vi "Digilens DLP Gen2 UI .vi"(11 "TopLevel In":refnum<class "TopLevel.lvclass">) -> (3 "TopLevel Out":refnum<class "TopLevel.lvclass">)   [LabVIEW 2022 SP3, in "TopLevel.lvclass"] (continued)
            n239 = call <vilib>:"Add State(s) to Queue__JKI_lib_State_Machine.vi"("State(s) in Front (\"\")"="UI: CheckConfigRequired\nUI: UpatePrinterPage" ("State(s) in Front (\"\")"), "State(s) in (\"\")"=w621) -> ("States Out"=w620:string)  [unwired: 13 in]
          }
          event User Event {
            (unwired) "Data: Verify Materials and Color planes" ("State(s) in Front (\"\")")
            n240 = event-data() -> ("Paths"=w660:T36, "ColorPaneMapping"=w659:T37)  [unwired: 1 in, 4 out]
            n241 = Bundle By Name(cluster=w663, "DLP2Config.Paths"=w660, "DLP2Config.ColorPaneMapping"=w659) -> (w661:T77)
            n242 = call <vilib>:"Add State(s) to Queue__JKI_lib_State_Machine.vi"("State(s) in (\"\")"=w666) -> ("States Out"=w665:string)  [unwired: 14 in]
          }
          event "Apply DLP GUI Config": Value Change {
            # "Note: Cannot be blocking"
            n243 = event-data() -> ()  [unwired: 1 in, 6 out]
            n244 = call-dynamic "ApplyDLP2GUIConfig_API.vi"("error in (no error)"=w668, "DLP GUI Config"="DLP GUI Config", "TopLevel in"=w670) -> ("error out"=w669:errorcluster, "TopLevel out"=w671:refnum<class "TopLevel.lvclass">)  [unwired: 7 in]
            n245 = call <vilib>:"Add State(s) to Queue__JKI_lib_State_Machine.vi"("State(s) in (\"\")"=w674) -> ("States Out"=w673:string)  [unwired: 14 in]
          }
          event "SAVE DLP Config": Value Change {
            n246 = event-data() -> ()  [unwired: 1 in, 6 out]
            n247 = Unbundle By Name(w685) -> ("TopLevel out"=w684:refnum<class "TopLevel.lvclass">, "DLP2Config"=w676:T35)
            n248 = call-dynamic "Write Digilens Config 2.vi"("error in (no error)"=w683, "MasterConfigurationDLPC2"=w676, "TopLevel in"=w684) -> ("error out"=w679:errorcluster, "TopLevel out"=w681:refnum<class "TopLevel.lvclass">)  [unwired: 7 in]
            n249 = property on="DLP GUI Config" class="Path"(error in=w679) -> (error out=w680:errorcluster, "Value"=w682:path)  [unwired: 1 in, 1 out]
            n250 = call-dynamic "SaveDLP2GUIConfig_API.vi"("error in (no error)"=w680, "DLP GUI Config"=w682, "TopLevel in"=w681) -> ("error out"=w678:errorcluster)  [unwired: 7 in, 1 out]
            n251 = Bundle By Name(cluster=w685, "DLP2ConfigLoaded"=w676, "ConfigSaveRequired"=FALSE) -> (w677:T77)
            n252 = call <vilib>:"Add State(s) to Queue__JKI_lib_State_Machine.vi"("State(s) in (\"\")"=w688) -> ("States Out"=w687:string)  [unwired: 14 in]
          }
          event "GetMat&Color": Value Change {
            n253 = event-data() -> ()  [unwired: 1 in, 6 out]
            n254 = call <vilib>:"Add State(s) to Queue__JKI_lib_State_Machine.vi"("State(s) in Front (\"\")"="Data: GetMaterialsAndColorPlanes" ("State(s) in Front (\"\")"), "State(s) in (\"\")"=w694) -> ("States Out"=w693:string)  [unwired: 13 in]
          }
          event User Event {
            n255 = event-data() -> ("PrintNo"=→"Print #":i32, "PrePurgePrintNo"=→"Counts":i32, "CalPrintNo"=→"CalPrint Counter":i32)  [unwired: 1 in, 7 out]
            n256 = call <vilib>:"Add State(s) to Queue__JKI_lib_State_Machine.vi"("State(s) in Front (\"\")"="UI: Update Stage Busy" ("State(s) in Front (\"\")"), "State(s) in (\"\")"=w703) -> ("States Out"=w702:string)  [unwired: 13 in]
          }
          event "Abort", "AbortPrinterOperation", "Abort 2": Value Change {
            n257 = event-data() -> ()  [unwired: 1 in, 6 out]
            n258 = Unbundle By Name(w718) -> ("TopLevel out"=w707:refnum<class "TopLevel.lvclass">, "Motor Controller"=w715:refnum<class "Motor Controller.lvclass">, "GIS Printer"=w709:refnum<class "GIS Printer.lvclass">)
            n259 = call-dynamic "Abort API.vi"("error in (no error)"=w705, "TopLevel in"=w707) -> ("error out"=w706:errorcluster)  [unwired: 8 in, 1 out]
            n260 = call "Generate Abort Event GIS Printer.vi"("error in (no error)"=w706, "GIS Printer in"=w709) -> ("error out"=w710:errorcluster, "GIS Printer out"=w708:refnum<class "GIS Printer.lvclass">)  [unwired: 8 in]
            n261 = disable-structure shown="Enabled" {
              disable-tunnel: "AbortPrint" ("Task ID") -> [w726 _]
              disable-tunnel: FALSE ("Wait (F)") -> [w725 _]
              disable-tunnel: [w724 w727] -> w712
              disable-tunnel: w708 -> [w723 _]
              disable-tunnel: w710 -> [w722 w727]
              frame Disabled {
                n262 = call "API_Abort.vi"("Wait (F)"=w725, "error in (no error)"=w722, "Task ID"=w726, "GIS Printer in"=w723) -> ("error out"=w724:errorcluster)  [unwired: 5 in, 2 out]
              }
              frame Enabled {
              }
            }
            n263 = call "API_AbortStage.vi"("Wait (F)"=FALSE, "error in (no error)"=w712, "Task ID"="AbortMotor", "Motor Controller in"=w715) -> ("error out"=w711:errorcluster)  [unwired: 5 in, 2 out]
            n264 = call <vilib>:"Add State(s) to Queue__JKI_lib_State_Machine.vi"("State(s) in Front (\"\")"="UI: Update Status>>Abort" ("State(s) in Front (\"\")"), "State(s) in (\"\")"=w721) -> ("States Out"=w720:string)  [unwired: 13 in]
          }
          event "Stage Abort": Value Change {
            n265 = event-data() -> ()  [unwired: 1 in, 6 out]
            n266 = Unbundle By Name(w733) -> ("Motor Controller"=w732:refnum<class "Motor Controller.lvclass">)  [unwired: 1 out]
            n267 = call "API_AbortStage.vi"("Wait (F)"=FALSE, "error in (no error)"=w728, "Task ID"="AbortMotor", "Motor Controller in"=w732) -> ("error out"=w729:errorcluster)  [unwired: 5 in, 2 out]
            n268 = call <vilib>:"Add State(s) to Queue__JKI_lib_State_Machine.vi"("State(s) in (\"\")"=w736) -> ("States Out"=w735:string)  [unwired: 14 in]
          }
          event Panel Close? {
            # "Discard the event because we'll close the front panel ourselves in Macro: Exit"
            n269 = event-data() -> ()  [unwired: 1 in, 1 out]
            n270 = event-data("Discard?"=TRUE) -> ()  [unwired: 1 in, 1 out]
            n271 = call <vilib>:"Add State(s) to Queue__JKI_lib_State_Machine.vi"("State(s) in Front (\"\")"="Macro: Exit", "State(s) in (\"\")"=w743) -> ("States Out"=w742:string)  [unwired: 13 in]
          }
          event "Exit": Value Change {
            n272 = event-data() -> ()  [unwired: 1 in, 6 out]
            n273 = Two Button Dialog(message="Are you sure you want to Exit the Application?", 2:"Exit" ("T button name (\"OK\")")) -> (T button?=w747:bool)  [unwired: 1 in]
            n274 = Select(t="Macro: Exit", s=w747, f="") -> (s? t:f=w744:string)
            n275 = call <vilib>:"Add State(s) to Queue__JKI_lib_State_Machine.vi"("State(s) in Front (\"\")"=w744, "State(s) in (\"\")"=w754) -> ("States Out"=w753:string)  [unwired: 13 in]
          }
          event User Event {
            n276 = event-data() -> ("Motor Controller Config Data"=w763:T41, "Motor Controller Data"=w762:cluster{"Enabled?":bool}, "Stage Move.Current Step"=→"Status":string, "Stage Move.Move Data"=w761:T43[], "Stage Busy?"=w755:bool)  [unwired: 1 in, 4 out]
            n277 = flat-sequence {
              tunnel: w755 -> [_]
              frame #0 {
              }
            }
            n278 = Unbundle By Name(w763) -> ("Current Position"=→"Position":i32, "Pulse_Per_mm"=→"Pulse/mm":i32, "PrePrint"=w771:dbl[])
            n279 = Unbundle By Name(w762) -> ()  [unwired: 1 out]
            n280 = Bundle By Name(cluster=w775, "Status.Motor Controller Config Data"=w763, "Status.Motor Controller Data"=w762) -> (w764:T77)
            n281 = for {
              tunnel: w761 -> [w784] mode=indexing
              tunnel: [w777] -> w759 mode=indexing
              n282 = Unbundle By Name(w784) -> ("Move.Index_mm"=w783:i32, "Move.Speed_mm_s"=w782:i32, "Status"=w779:T44)
              n283 = Format Into String(w783) -> (resulting string=w781:string)  [unwired: 3 in, 1 out]
              n284 = Format Into String(w782) -> (resulting string=w780:string)  [unwired: 3 in, 1 out]
              n285 = Format Into String(w779) -> (resulting string=w778:string)  [unwired: 3 in, 1 out]
              n286 = Build Array(w781, w780, w778) -> (w777:string[])
            }
            n287 = Index Array(array=w771) -> (element #1=→"H1":dbl, element #2=→"H 2":dbl, element #3=→"H 3":dbl, element #4=→"H 4":dbl, element #5=→"H 5":dbl, element #6=→"H 6":dbl)  [unwired: 6 in]
            n288 = property on="Stage Move Status" class="MCListbox (strict)"("ItemNames"=w759) -> ()  [unwired: 2 in, 2 out]
            n289 = call <vilib>:"Add State(s) to Queue__JKI_lib_State_Machine.vi"("State(s) in Front (\"\")"="UI: Update Stage Busy", "State(s) in (\"\")"=w757) -> ("States Out"=w758:string)  [unwired: 13 in]
          }
          event User Event {
            n290 = event-data() -> ("UsrEvtRef"=w790:refnum<user-event>)  [unwired: 1 in, 3 out]
            n291 = Flush Event Queue(0:w791, 2:w790, 3:w786, 5:1 ("keep most recent")) -> (8:w788:refnum<event-registration>, 11:w787:errorcluster)  [unwired: 2 in, 1 out]
            n292 = call <vilib>:"Add State(s) to Queue__JKI_lib_State_Machine.vi"("State(s) in Front (\"\")"="DI: Get ICP2 DI Status\nDO: Set ICP1-DO Status in UI\nDO: Set ICP2-DO Status in UI\nAI: Get ICP1 AI Status\nAO: Set ICP1-AO Status in UI\nAO: Set ICP2-AO Status in UI" ("State(s) in Front (\"\")"), "State(s) in (\"\")"=w792) -> ("States Out"=w793:string)  [unwired: 13 in]
          }
          event Value Change {
            n293 = event-data() -> ()  [unwired: 1 in, 6 out]
            n294 = case shown="True" "Enable Disable" {
              tunnel: [Motor_Controller_Parameter-Set."Enable Servo" ("Motor Controller Parameter") Motor_Controller_Parameter-Set."Disable Servo" ("Motor Controller Parameter")] -> w807
              tunnel: [1 ("value") 0 ("value")] -> w804
              frame True {
              }
              frame False {
              }
            }
            n295 = Bundle By Name(cluster=T20 {"Motor Controller Parameter"=enum."Print Speed", "value"=0} ("SetExplicitMessage API Data"), "Motor Controller Parameter"=w807, "value"=w804) -> (w806:T20)
            n296 = Unbundle By Name(w801) -> ("Motor Controller"=w812:refnum<class "Motor Controller.lvclass">)
            n297 = Bundle By Name(cluster=T23 {"Command"=enum."GetExplicitMessage", "Arguments"="", "Data"=variant} ("API Command Cluster"), "Command"=API_Command_Enum."SetExplicitMessage", "Data"=w806) -> (w805:T23)
            n298 = call-dynamic "GenerateAPIEvent_Motor Controller.vi"("error in (no error)"=w811, "API Command Cluster"=w805, "Motor Controller In"=w812) -> ("error out"=w798:errorcluster)  [unwired: 6 in, 2 out]
            n299 = Unbundle By Name(w801) -> ("DAQ"=w802:refnum<class "DAQ.lvclass">)
            n300 = Format Into String(format string="%s", ICP1-D0_Channel_Names."Servo ON" ("DO Channel")) -> (resulting string=w800:string)  [unwired: 2 in, 1 out]
            n301 = call "Set DO State (manual mode).vi"("error in (no error)"=w798, "State"="Enable Disable", "DO IOName"=w800, "DAQ"=w802) -> ("error out"=w797:errorcluster)  [unwired: 6 in, 1 out]
          }
          event "5Pass": Value Change {
            n302 = event-data() -> ()  [unwired: 1 in, 6 out]
            n303 = Bundle By Name(cluster=T20 {"Motor Controller Parameter"=enum."Print Speed", "value"=0} ("SetExplicitMessage API Data"), "Motor Controller Parameter"=Motor_Controller_Parameter-Set."PR Path", "value"=20) -> (w821:T20)
            n304 = Unbundle By Name(w829) -> ("Motor Controller"=w828:refnum<class "Motor Controller.lvclass">)
            n305 = Bundle By Name(cluster=T23 {"Command"=enum."GetExplicitMessage", "Arguments"="", "Data"=variant} ("API Command Cluster"), "Command"=API_Command_Enum."SetExplicitMessage", "Data"=w821) -> (w820:T23)
            n306 = call-dynamic "GenerateAPIEvent_Motor Controller.vi"("error in (no error)"=w826, "API Command Cluster"=w820, "Motor Controller In"=w828) -> ("error out"=w827:errorcluster)  [unwired: 6 in, 2 out]
          }
          event "10Pass": Value Change {
            n307 = event-data() -> ()  [unwired: 1 in, 6 out]
            n308 = Bundle By Name(cluster=T20 {"Motor Controller Parameter"=enum."Print Speed", "value"=0} ("SetExplicitMessage API Data"), "Motor Controller Parameter"=Motor_Controller_Parameter-Set."PR Path", "value"=30) -> (w834:T20)
            n309 = Unbundle By Name(w842) -> ("Motor Controller"=w841:refnum<class "Motor Controller.lvclass">)
            n310 = Bundle By Name(cluster=T23 {"Command"=enum."GetExplicitMessage", "Arguments"="", "Data"=variant} ("API Command Cluster"), "Command"=API_Command_Enum."SetExplicitMessage", "Data"=w834) -> (w833:T23)
            n311 = call-dynamic "GenerateAPIEvent_Motor Controller.vi"("error in (no error)"=w839, "API Command Cluster"=w833, "Motor Controller In"=w841) -> ("error out"=w840:errorcluster)  [unwired: 6 in, 2 out]
          }
          event Value Change {
            n312 = event-data() -> ("CtlRef"=w847:refnum<vi>)  [unwired: 1 in, 5 out]
            n313 = property class="Bool"(reference=w847) -> ("Label.Text"=w846:string)  [unwired: 1 in, 2 out]
            n314 = case shown="\"Head6\"" w846 {
              tunnel: [Motor_Controller_Parameter-Set."Move Stage to Under PH1" ("Motor Controller Parameter") Motor_Controller_Parameter-Set."Move Stage to Under PH1" ("Motor Controller Parameter") Motor_Controller_Parameter-Set."Move Stage to Under PH2" ("Motor Controller Parameter") Motor_Controller_Parameter-Set."Move Stage to Under PH2" ("Motor Controller Parameter") Motor_Controller_Parameter-Set."Move Stage to Under PH3" ("Motor Controller Parameter") Motor_Controller_Parameter-Set."Move Stage to Under PH3" ("Motor Controller Parameter") Motor_Controller_Parameter-Set."Move Stage to Under PH4" ("Motor Controller Parameter") Motor_Controller_Parameter-Set."Move Stage to Under PH4" ("Motor Controller Parameter") Motor_Controller_Parameter-Set."Move Stage to Under PH5" ("Motor Controller Parameter") Motor_Controller_Parameter-Set."Move Stage to Under PH5" ("Motor Controller Parameter") Motor_Controller_Parameter-Set."Move Stage to Under PH6" ("Motor Controller Parameter") Motor_Controller_Parameter-Set."Move Stage to Under PH6" ("Motor Controller Parameter")] -> w849
              tunnel: [11 ("value") 4 ("value") 12 ("value") 5 ("value") 13 ("value") 6 ("value") 14 ("value") 7 ("value") 15 ("value") 8 ("value") 16 ("value") 9 ("value")] -> w848
              frame "Head1", Default {
              }
              frame "PurgeMove H1" {
              }
              frame "Head2" {
              }
              frame "PurgeMove H2" {
              }
              frame "Head3" {
              }
              frame "PurgeMove H3" {
              }
              frame "Head4" {
              }
              frame "PurgeMove H4" {
              }
              frame "Head5" {
              }
              frame "PurgeMove H5" {
              }
              frame "Head6" {
              }
              frame "PurgeMove H6" {
              }
            }
            n315 = Bundle By Name(cluster=T20 {"Motor Controller Parameter"=enum."Move Stage to Under PH1", "value"=11} ("SetExplicitMessage API Data"), "value"=w848, "Motor Controller Parameter"=w849) -> (w845:T20)
            n316 = Unbundle By Name(w853) -> ("Motor Controller"=w857:refnum<class "Motor Controller.lvclass">)
            n317 = Bundle By Name(cluster=T23 {"Command"=enum."GetExplicitMessage", "Arguments"="", "Data"=variant} ("API Command Cluster"), "Command"=API_Command_Enum."SetExplicitMessage", "Data"=w845) -> (w854:T23)
            n318 = call-dynamic "GenerateAPIEvent_Motor Controller.vi"("error in (no error)"=w851, "API Command Cluster"=w854, "Motor Controller In"=w857) -> ("error out"=w852:errorcluster)  [unwired: 6 in, 2 out]
          }
          event "Heater-1 Off 2": Value Change {
            n319 = event-data() -> ("NewVal"=w884:bool)  [unwired: 1 in, 5 out]
            n320 = Bundle By Name(cluster=w891, "Heater Enable.HeaterEnblHead"=PrinterHeads--Enum."1" ("Heater Enable.Head"), "Heater Enable.Enable"=w884, "PersistentData.HeatEnable.Heater-1 Off"=w884) -> (w889:T77)
            n321 = call <vilib>:"Add State(s) to Queue__JKI_lib_State_Machine.vi"("State(s) in Front (\"\")"="Heater: Enable Disable\nData: Write to Persistent File", "State(s) in (\"\")"=w886) -> ("States Out"=w887:string)  [unwired: 13 in]
          }
          event "Heater-2 Off 2": Value Change {
            n322 = event-data() -> ("NewVal"=w893:bool)  [unwired: 1 in, 5 out]
            n323 = Bundle By Name(cluster=w900, "Heater Enable.HeaterEnblHead"=PrinterHeads--Enum."2" ("Heater Enable.Head"), "Heater Enable.Enable"=w893, "PersistentData.HeatEnable.Heater-2 Off"=w893) -> (w898:T77)
            n324 = call <vilib>:"Add State(s) to Queue__JKI_lib_State_Machine.vi"("State(s) in Front (\"\")"="Heater: Enable Disable\nData: Write to Persistent File", "State(s) in (\"\")"=w895) -> ("States Out"=w896:string)  [unwired: 13 in]
          }
          event "Heater-3 Off 2": Value Change {
            n325 = event-data() -> ("NewVal"=w902:bool)  [unwired: 1 in, 5 out]
            n326 = Bundle By Name(cluster=w909, "Heater Enable.HeaterEnblHead"=PrinterHeads--Enum."3" ("Heater Enable.Head"), "Heater Enable.Enable"=w902, "PersistentData.HeatEnable.Heater-3 Off"=w902) -> (w907:T77)
            n327 = call <vilib>:"Add State(s) to Queue__JKI_lib_State_Machine.vi"("State(s) in Front (\"\")"="Heater: Enable Disable\nData: Write to Persistent File", "State(s) in (\"\")"=w904) -> ("States Out"=w905:string)  [unwired: 13 in]
          }
          event "Heater-4 Off 2": Value Change {
            n328 = event-data() -> ("NewVal"=w911:bool)  [unwired: 1 in, 5 out]
            n329 = Bundle By Name(cluster=w918, "Heater Enable.HeaterEnblHead"=PrinterHeads--Enum."4" ("Heater Enable.Head"), "Heater Enable.Enable"=w911, "PersistentData.HeatEnable.Heater-4 Off"=w911) -> (w916:T77)
            n330 = call <vilib>:"Add State(s) to Queue__JKI_lib_State_Machine.vi"("State(s) in Front (\"\")"="Heater: Enable Disable\nData: Write to Persistent File", "State(s) in (\"\")"=w913) -> ("States Out"=w914:string)  [unwired: 13 in]
          }
          event "Heater-5 Off 2": Value Change {
            n331 = event-data() -> ("NewVal"=w920:bool)  [unwired: 1 in, 5 out]
            n332 = Bundle By Name(cluster=w927, "Heater Enable.HeaterEnblHead"=PrinterHeads--Enum."5" ("Heater Enable.Head"), "Heater Enable.Enable"=w920, "PersistentData.HeatEnable.Heater-5 Off"=w920) -> (w925:T77)
            n333 = call <vilib>:"Add State(s) to Queue__JKI_lib_State_Machine.vi"("State(s) in Front (\"\")"="Heater: Enable Disable\nData: Write to Persistent File", "State(s) in (\"\")"=w922) -> ("States Out"=w923:string)  [unwired: 13 in]
          }
          event "Heater-6 Off 2": Value Change {
            n334 = event-data() -> ("NewVal"=w929:bool)  [unwired: 1 in, 5 out]
            n335 = Bundle By Name(cluster=w936, "Heater Enable.HeaterEnblHead"=PrinterHeads--Enum."6" ("Heater Enable.Head"), "Heater Enable.Enable"=w929, "PersistentData.HeatEnable.Heater-6 Off"=w929) -> (w934:T77)
            n336 = call <vilib>:"Add State(s) to Queue__JKI_lib_State_Machine.vi"("State(s) in Front (\"\")"="Heater: Enable Disable\nData: Write to Persistent File", "State(s) in (\"\")"=w931) -> ("States Out"=w932:string)  [unwired: 13 in]
          }
          event "Head Print Command": Value Change {
            n337 = event-data() -> ()  [unwired: 1 in, 6 out]
            n338 = local write "Head Print Command"(FALSE ("Head Print Command")) -> ()
            n339 = Unbundle By Name(w963) -> ("TopLevel out"=w947:refnum<class "TopLevel.lvclass">, "CalibrationPrints.CellPrintRecipe.CellPrint"=w955:T81)
            n340 = property on="PrintHead Number" class="Ring (strict)"() -> ("RingText.Text"=w949:string)  [unwired: 2 in, 2 out]
            n341 = Decimal String To Number(string=w949) -> (number=w945:i32)  [unwired: 2 in, 1 out]
            n342 = for {
              tunnel: w955 -> [w975] mode=indexing
              tunnel: w945 -> [w973]
              tunnel: [w972] -> w951
              stop <- w971 stop-if-true
              n343 = Unbundle By Name(w975) -> ("#attributes"=w972:T82, "#attributes.Head"=w974:i32)
              n344 = Equal?(x=w974, y=w973) -> (x = y?=w971:bool)
            }
            n345 = Unbundle By Name(w951) -> ("PrintPass"=w950:i32, "PrintImageFile"=w954:string, "EncoderSource"=w953:string, "PrintGoSource"=w952:string)
            n346 = To Unsigned Byte Integer(number=w950) -> (unsigned 8bit integer=w944:u8)
            n347 = case shown="2" w945 {
              tunnel: [PrinterHeads--Enum."-1" ("Head") PrinterHeads--Enum."1" ("Head") PrinterHeads--Enum."2" ("Head") PrinterHeads--Enum."3" ("Head") PrinterHeads--Enum."4" ("Head") PrinterHeads--Enum."5" ("Head") PrinterHeads--Enum."6" ("Head")] -> w946
              frame 0, Default {
              }
              frame 1 {
              }
              frame 2 {
              }
              frame 3 {
              }
              frame 4 {
              }
              frame 5 {
              }
              frame 6 {
              }
            }
            n348 = Bundle By Name(cluster=T24 {"PrintImageFile"="", "PrintPass"=1, "EncoderSource"="", "PrintGoSource"="", "Head"=enum."1"} ("#attributes"), "PrintPass"=w944, "PrintImageFile"=w954, "EncoderSource"=w953, "PrintGoSource"=w952) -> (w957:T24)
            n349 = Multiply(x=w944, y=10000) -> (x*y=w941:i32)
            n350 = Add(x=w941, y=30000) -> (x+y=w940:i32)
            n351 = Bundle By Name(cluster=w957, "Head"=w946) -> (w956:T24)
            n352 = call-dynamic "HeadPrint API.vi"("Timeout (ms)"=w940, "error in (no error)"=w960, "HeadPrint Data"=w956, "TopLevel in"=w947) -> ("error out"=w961:errorcluster)  [unwired: 6 in, 1 out]
            n353 = call <vilib>:"Add State(s) to Queue__JKI_lib_State_Machine.vi"("State(s) in Front (\"\")"="UI: Update Status>>Running Calibration Prints" ("State(s) in Front (\"\")"), "State(s) in (\"\")"=w959) -> ("States Out"=w958:string)  [unwired: 13 in]
          }
          event "Head1 Temp 1": Value Change {
            n354 = event-data() -> ("OldVal"=w985:string, "NewVal"=w988:string)  [unwired: 1 in, 4 out]
            n355 = Scan From String(format string="%f/%#.f", input string=w988) -> (error out=w986:errorcluster, output 2=w984:dbl)  [unwired: 5 in, 2 out]
            n356 = case shown="No Error" w986 {
              tunnel: w985 -> [_ w998]
              tunnel: w984 -> [w993 _]
              tunnel: w982 -> [w995 w997]
              tunnel: [w994 w997] -> w983
              tunnel: w978 -> [w991 _]
              tunnel: w976 -> [w990 w996]
              tunnel: [w989 w996] -> w977
              frame No Error {
                n357 = Bundle By Name(cluster=w995, "Head Temp.Head 1.Target"=w993) -> (w994:T77)
                n358 = call-dynamic "SetHeadHeaterTemperature API.vi"("error in (no error)"=w990, "SetPoint (deg)"=w993, "Head"=PrinterHeads--Enum."1", "TopLevel in"=w991) -> ("error out"=w989:errorcluster)  [unwired: 6 in, 1 out]
              }
              frame Error {
                n359 = local write "Head1 Temp 1"(w998) -> ()
              }
            }
            n360 = call <vilib>:"Add State(s) to Queue__JKI_lib_State_Machine.vi"("State(s) in Front (\"\")"="UI: Display Heater Temperature", "State(s) in (\"\")"=w980) -> ("States Out"=w981:string)  [unwired: 13 in]
          }
          event "Head2 Temp 1": Value Change {
            n361 = event-data() -> ("OldVal"=w1008:string, "NewVal"=w1011:string)  [unwired: 1 in, 4 out]
            n362 = Scan From String(format string="%f/%#.f", input string=w1011) -> (error out=w1009:errorcluster, output 2=w1007:dbl)  [unwired: 5 in, 2 out]
            n363 = case shown="Error .." w1009 {
              tunnel: w1008 -> [_ w1021]
              tunnel: w1007 -> [w1016 _]
              tunnel: w1005 -> [w1018 w1020]
              tunnel: [w1017 w1020] -> w1006
              tunnel: w1001 -> [w1014 _]
              tunnel: w999 -> [w1013 w1019]
              tunnel: [w1012 w1019] -> w1000
              frame No Error {
                n364 = Bundle By Name(cluster=w1018, "Head Temp.Head 1.Target"=w1016) -> (w1017:T77)
                n365 = call-dynamic "SetHeadHeaterTemperature API.vi"("error in (no error)"=w1013, "SetPoint (deg)"=w1016, "Head"=PrinterHeads--Enum."2", "TopLevel in"=w1014) -> ("error out"=w1012:errorcluster)  [unwired: 6 in, 1 out]
              }
              frame Error {
                n366 = local write "Head2 Temp 1"(w1021) -> ()
              }
            }
            n367 = call <vilib>:"Add State(s) to Queue__JKI_lib_State_Machine.vi"("State(s) in Front (\"\")"="UI: Display Heater Temperature", "State(s) in (\"\")"=w1003) -> ("States Out"=w1004:string)  [unwired: 13 in]
          }
          event "Head3 Temp 1": Value Change {
            n368 = event-data() -> ("OldVal"=w1031:string, "NewVal"=w1034:string)  [unwired: 1 in, 4 out]
            n369 = Scan From String(format string="%f/%#.f", input string=w1034) -> (error out=w1032:errorcluster, output 2=w1030:dbl)  [unwired: 5 in, 2 out]
            n370 = case shown="No Error" w1032 {
              tunnel: w1031 -> [_ w1044]
              tunnel: w1030 -> [w1039 _]
              tunnel: w1028 -> [w1041 w1043]
              tunnel: [w1040 w1043] -> w1029
              tunnel: w1024 -> [w1037 _]
              tunnel: w1022 -> [w1036 w1042]
              tunnel: [w1035 w1042] -> w1023
              frame No Error {
                n371 = Bundle By Name(cluster=w1041, "Head Temp.Head 1.Target"=w1039) -> (w1040:T77)
                n372 = call-dynamic "SetHeadHeaterTemperature API.vi"("error in (no error)"=w1036, "SetPoint (deg)"=w1039, "Head"=PrinterHeads--Enum."3", "TopLevel in"=w1037) -> ("error out"=w1035:errorcluster)  [unwired: 6 in, 1 out]
              }
              frame Error {
                n373 = local write "Head3 Temp 1"(w1044) -> ()
              }
            }
            n374 = call <vilib>:"Add State(s) to Queue__JKI_lib_State_Machine.vi"("State(s) in Front (\"\")"="UI: Display Heater Temperature", "State(s) in (\"\")"=w1026) -> ("States Out"=w1027:string)  [unwired: 13 in]
          }
          event "Head4 Temp 1": Value Change {
            n375 = event-data() -> ("OldVal"=w1054:string, "NewVal"=w1057:string)  [unwired: 1 in, 4 out]
            n376 = Scan From String(format string="%f/%#.f", input string=w1057) -> (error out=w1055:errorcluster, output 2=w1053:dbl)  [unwired: 5 in, 2 out]
            n377 = case shown="Error .." w1055 {
              tunnel: w1054 -> [_ w1067]
              tunnel: w1053 -> [w1062 _]
              tunnel: w1051 -> [w1064 w1066]
              tunnel: [w1063 w1066] -> w1052
              tunnel: w1047 -> [w1060 _]
              tunnel: w1045 -> [w1059 w1065]
              tunnel: [w1058 w1065] -> w1046
              frame No Error {
                n378 = Bundle By Name(cluster=w1064, "Head Temp.Head 1.Target"=w1062) -> (w1063:T77)
                n379 = call-dynamic "SetHeadHeaterTemperature API.vi"("error in (no error)"=w1059, "SetPoint (deg)"=w1062, "Head"=PrinterHeads--Enum."4", "TopLevel in"=w1060) -> ("error out"=w1058:errorcluster)  [unwired: 6 in, 1 out]
              }
              frame Error {
                n380 = local write "Head4 Temp 1"(w1067) -> ()
              }
            }
            n381 = call <vilib>:"Add State(s) to Queue__JKI_lib_State_Machine.vi"("State(s) in Front (\"\")"="UI: Display Heater Temperature", "State(s) in (\"\")"=w1049) -> ("States Out"=w1050:string)  [unwired: 13 in]
          }
          event "Head5 Temp 1": Value Change {
            n382 = event-data() -> ("OldVal"=w1077:string, "NewVal"=w1080:string)  [unwired: 1 in, 4 out]
            n383 = Scan From String(format string="%f/%#.f", input string=w1080) -> (error out=w1078:errorcluster, output 2=w1076:dbl)  [unwired: 5 in, 2 out]
            n384 = case shown="Error .." w1078 {
              tunnel: w1077 -> [_ w1090]
              tunnel: w1076 -> [w1085 _]
              tunnel: w1074 -> [w1087 w1089]
              tunnel: [w1086 w1089] -> w1075
              tunnel: w1070 -> [w1083 _]
              tunnel: w1068 -> [w1082 w1088]
              tunnel: [w1081 w1088] -> w1069
              frame No Error {
                n385 = Bundle By Name(cluster=w1087, "Head Temp.Head 1.Target"=w1085) -> (w1086:T77)
                n386 = call-dynamic "SetHeadHeaterTemperature API.vi"("error in (no error)"=w1082, "SetPoint (deg)"=w1085, "Head"=PrinterHeads--Enum."5", "TopLevel in"=w1083) -> ("error out"=w1081:errorcluster)  [unwired: 6 in, 1 out]
              }
              frame Error {
                n387 = local write "Head5 Temp 1"(w1090) -> ()
              }
            }
            n388 = call <vilib>:"Add State(s) to Queue__JKI_lib_State_Machine.vi"("State(s) in Front (\"\")"="UI: Display Heater Temperature", "State(s) in (\"\")"=w1072) -> ("States Out"=w1073:string)  [unwired: 13 in]
          }
          event "Head6 Temp 1": Value Change {
            n389 = event-data() -> ("OldVal"=w1100:string, "NewVal"=w1103:string)  [unwired: 1 in, 4 out]
            n390 = Scan From String(format string="%f/%#.f", input string=w1103) -> (error out=w1101:errorcluster, output 2=w1099:dbl)  [unwired: 5 in, 2 out]
            n391 = case shown="Error .." w1101 {
              tunnel: w1100 -> [_ w1113]
              tunnel: w1099 -> [w1108 _]
              tunnel: w1097 -> [w1110 w1112]
              tunnel: [w1109 w1112] -> w1098
              tunnel: w1093 -> [w1106 _]
              tunnel: w1091 -> [w1105 w1111]
              tunnel: [w1104 w1111] -> w1092
              frame No Error {
                n392 = Bundle By Name(cluster=w1110, "Head Temp.Head 1.Target"=w1108) -> (w1109:T77)
                n393 = call-dynamic "SetHeadHeaterTemperature API.vi"("error in (no error)"=w1105, "SetPoint (deg)"=w1108, "Head"=PrinterHeads--Enum."6", "TopLevel in"=w1106) -> ("error out"=w1104:errorcluster)  [unwired: 6 in, 1 out]
              }
              frame Error {
                n394 = local write "Head6 Temp 1"(w1113) -> ()
              }
            }
            n395 = call <vilib>:"Add State(s) to Queue__JKI_lib_State_Machine.vi"("State(s) in Front (\"\")"="UI: Display Heater Temperature", "State(s) in (\"\")"=w1095) -> ("States Out"=w1096:string)  [unwired: 13 in]
          }
          event "Home", "Home 3": Value Change {
            n396 = event-data() -> ()  [unwired: 1 in, 6 out]
            n397 = Unbundle By Name(w1118) -> ("Motor Controller"=w1119:refnum<class "Motor Controller.lvclass">)
            n398 = call "API_HomeStage.vi"("Timeout (ms)"=u32 600000, "Wait (F)"=FALSE, "error in (no error)"=w1116, "Motor Controller in"=w1119) -> ("error out"=w1117:errorcluster)  [unwired: 5 in, 2 out]
          }
          event Value Change {
            n399 = event-data() -> ()  [unwired: 1 in, 6 out]
            n400 = Unbundle By Name(w1128) -> ("Motor Controller"=w1132:refnum<class "Motor Controller.lvclass">)  [unwired: 1 out]
            n401 = Bundle By Name(cluster=T20 {"Motor Controller Parameter"=enum."Write Speed", "value"=0} ("SetExplicitMessage API Data"), "Motor Controller Parameter"=Motor_Controller_Parameter-Set."Return Stage to 0", "value"=0) -> (w1123:T20)
            n402 = Bundle By Name(cluster=T23 {"Command"=enum."GetExplicitMessage", "Arguments"="", "Data"=variant} ("API Command Cluster"), "Command"=API_Command_Enum."SetExplicitMessage", "Data"=w1123) -> (w1129:T23)
            n403 = call-dynamic "GenerateAPIEvent_Motor Controller.vi"("error in (no error)"=w1126, "API Command Cluster"=w1129, "Motor Controller In"=w1132) -> ("error out"=w1127:errorcluster)  [unwired: 6 in, 2 out]
          }
          event Value Change {
            n404 = event-data() -> ()  [unwired: 1 in, 6 out]
            n405 = Unbundle By Name(w1137) -> ("Motor Controller"=w1138:refnum<class "Motor Controller.lvclass">)  [unwired: 1 out]
            n406 = call "Laminate API.vi"("error in (no error)"=w1135, "Motor Controller in"=w1138) -> ("error out"=w1136:errorcluster)  [unwired: 7 in, 2 out]
          }
          event Value Change {
            # "Conversion done in SendLVEthIP_ExplicitMessage.vi"
            n407 = event-data() -> ()  [unwired: 1 in, 6 out]
            n408 = Unbundle By Name(w1169) -> ("Motor Controller"=w1159:refnum<class "Motor Controller.lvclass">)
            n409 = disable-structure shown="Enabled" {
              disable-tunnel: "Speed" -> [w1183 w1188]
              disable-tunnel: [w1182 w1188] -> w1153
              frame Disabled {
                n410 = Multiply(x=w1183, y=60 ("x")) -> (x*y=w1187:i32)
                n411 = Divide(x=w1187, y=12.7) -> (x/y=w1185:dbl)
                n412 = To Long Integer(number=w1185) -> (32bit integer=w1182:i32)
              }
              frame Enabled {
              }
            }
            n413 = local write "Go"(FALSE ("Go To")) -> ()
            n414 = Bundle By Name(cluster=T20 {"Motor Controller Parameter"=enum."Write Speed", "value"=0} ("SetExplicitMessage API Data"), "Motor Controller Parameter"=Motor_Controller_Parameter-Set."Write Speed", "value"=w1153) -> (w1165:T20)
            n415 = Bundle By Name(cluster=T23 {"Command"=enum."GetExplicitMessage", "Arguments"="", "Data"=variant} ("API Command Cluster"), "Command"=API_Command_Enum."SetExplicitMessage", "Data"=w1165) -> (w1162:T23)
            n416 = disable-structure shown="Disabled" {
              disable-tunnel: [w1177 w1181] -> w1152
              disable-tunnel: "GoTo" -> [w1175 w1181]
              frame Disabled {
                n417 = Divide(x=w1175, y=12.7) -> (x/y=w1180:dbl)
                n418 = Multiply(x=w1180, y=100000.0 ("x")) -> (x*y=w1178:dbl)
                n419 = To Long Integer(number=w1178) -> (32bit integer=w1177:i32)
              }
              frame Enabled {
              }
            }
            n420 = call-dynamic "GenerateAPIEvent_Motor Controller.vi"("error in (no error)"=w1156, "API Command Cluster"=w1162, "Motor Controller In"=w1159) -> ("error out"=w1157:errorcluster, "Motor Controller out"=w1158:refnum<class "Motor Controller.lvclass">)  [unwired: 6 in, 1 out]
            n421 = Bundle By Name(cluster=T20 {"Motor Controller Parameter"=enum."Write Speed", "value"=0} ("SetExplicitMessage API Data"), "Motor Controller Parameter"=Motor_Controller_Parameter-Set."Write Index", "value"=w1152) -> (w1166:T20)
            n422 = Bundle By Name(cluster=T20 {"Motor Controller Parameter"=enum."Write Speed", "value"=0} ("SetExplicitMessage API Data"), "Motor Controller Parameter"=Motor_Controller_Parameter-Set."PR Path", "value"=10) -> (w1150:T20)
            n423 = Bundle By Name(cluster=T23 {"Command"=enum."GetExplicitMessage", "Arguments"="", "Data"=variant} ("API Command Cluster"), "Command"=API_Command_Enum."SetExplicitMessage", "Data"=w1166) -> (w1170:T23)
            n424 = call-dynamic "GenerateAPIEvent_Motor Controller.vi"("error in (no error)"=w1157, "API Command Cluster"=w1170, "Motor Controller In"=w1158) -> ("error out"=w1142:errorcluster, "Motor Controller out"=w1143:refnum<class "Motor Controller.lvclass">)  [unwired: 6 in, 1 out]
            n425 = Bundle By Name(cluster=T23 {"Command"=enum."GetExplicitMessage", "Arguments"="", "Data"=variant} ("API Command Cluster"), "Command"=API_Command_Enum."SetExplicitMessage", "Data"=w1150) -> (w1147:T23)
            n426 = call-dynamic "GenerateAPIEvent_Motor Controller.vi"("error in (no error)"=w1142, "API Command Cluster"=w1147, "Motor Controller In"=w1143) -> ("error out"=w1141:errorcluster)  [unwired: 6 in, 2 out]
          }
          event "Jog (+)", "Jog (+) 1", "Jog (+) 2": Value Change {
            n427 = event-data() -> ("NewVal"=w1189:bool)  [unwired: 1 in, 5 out]
            n428 = Unbundle By Name(w1207) -> ("Motor Controller"=w1196:refnum<class "Motor Controller.lvclass">)
            n429 = property on="Jog Speed" class="DigNum (strict)"(error in=w1191) -> (error out=w1192:errorcluster, "Value"=w1190:i32)  [unwired: 1 in, 1 out]
            n430 = Select(t=4998, s=w1189, f=0) -> (s? t:f=w1198:i32)
            n431 = call "SetJogSpeed.vi"("Timeout (ms)"=u32 1000, "error in (no error)"=w1192, "Jog Speed"=w1190, "Motor Controller in"=w1196) -> ("error out"=w1193:errorcluster, "Motor Controller out"=w1195:refnum<class "Motor Controller.lvclass">)  [unwired: 6 in]
            n432 = Bundle By Name(cluster=T20 {"Motor Controller Parameter"=enum."Write Speed", "value"=0} ("SetExplicitMessage API Data"), "Motor Controller Parameter"=Motor_Controller_Parameter-Set."Jog Speed", "value"=w1198) -> (w1206:T20)
            n433 = Bundle By Name(cluster=T23 {"Command"=enum."GetExplicitMessage", "Arguments"="", "Data"=variant} ("API Command Cluster"), "Command"=API_Command_Enum."SetExplicitMessage", "Data"=w1206) -> (w1203:T23)
            n434 = call-dynamic "GenerateAPIEvent_Motor Controller.vi"("error in (no error)"=w1193, "API Command Cluster"=w1203, "Motor Controller In"=w1195) -> ("error out"=w1197:errorcluster)  [unwired: 6 in, 2 out]
          }
          event "Print (+)": Value Change {
            n435 = event-data() -> ()  [unwired: 1 in, 6 out]
            n436 = Select(t=4998, s="Print (+)", f=0) -> (s? t:f=w1212:i32)
            n437 = Unbundle By Name(w1223) -> ("Motor Controller"=w1216:refnum<class "Motor Controller.lvclass">)
            n438 = Bundle By Name(cluster=T20 {"Motor Controller Parameter"=enum."Write Speed", "value"=0} ("SetExplicitMessage API Data"), "Motor Controller Parameter"=Motor_Controller_Parameter-Set."Write Speed", "value"=w1212) -> (w1222:T20)
            n439 = local write "Print Speed"(w1212) -> ()
            n440 = Bundle By Name(cluster=T23 {"Command"=enum."GetExplicitMessage", "Arguments"="", "Data"=variant} ("API Command Cluster"), "Command"=API_Command_Enum."SetExplicitMessage", "Data"=w1222) -> (w1219:T23)
            n441 = call-dynamic "GenerateAPIEvent_Motor Controller.vi"("error in (no error)"=w1215, "API Command Cluster"=w1219, "Motor Controller In"=w1216) -> ("error out"=w1211:errorcluster)  [unwired: 6 in, 2 out]
          }
          event "Jog Speed": Value Change {
            n442 = event-data() -> ()  [unwired: 1 in, 6 out]
            n443 = Unbundle By Name(w1230) -> ("Motor Controller"=w1229:refnum<class "Motor Controller.lvclass">)
            n444 = call "SetJogSpeed.vi"("error in (no error)"=w1228, "Jog Speed"="Jog Speed", "Motor Controller in"=w1229) -> ("error out"=w1227:errorcluster)  [unwired: 7 in, 1 out]
          }
          event "Print Speed": Value Change {
            n445 = event-data() -> ()  [unwired: 1 in, 6 out]
            n446 = Unbundle By Name(w1243) -> ("Motor Controller"=w1236:refnum<class "Motor Controller.lvclass">)
            n447 = Bundle By Name(cluster=T20 {"Motor Controller Parameter"=enum."Write Speed", "value"=0} ("SetExplicitMessage API Data"), "Motor Controller Parameter"=Motor_Controller_Parameter-Set."Write Speed", "value"="Print Speed") -> (w1242:T20)
            n448 = Bundle By Name(cluster=T23 {"Command"=enum."GetExplicitMessage", "Arguments"="", "Data"=variant} ("API Command Cluster"), "Command"=API_Command_Enum."SetExplicitMessage", "Data"=w1242) -> (w1239:T23)
            n449 = call-dynamic "GenerateAPIEvent_Motor Controller.vi"("error in (no error)"=w1235, "API Command Cluster"=w1239, "Motor Controller In"=w1236) -> ("error out"=w1234:errorcluster)  [unwired: 6 in, 2 out]
          }
          event "Jog (-)", "Jog (-) 1", "Jog (-) 2": Value Change {
            n450 = event-data() -> ("NewVal"=w1246:bool)  [unwired: 1 in, 5 out]
            n451 = property on="Jog Speed" class="DigNum (strict)"(error in=w1247) -> (error out=w1253:errorcluster, "Value"=w1252:i32)  [unwired: 1 in, 1 out]
            n452 = Unbundle By Name(w1264) -> ("Motor Controller"=w1250:refnum<class "Motor Controller.lvclass">)
            n453 = Select(t=4999, s=w1246, f=0) -> (s? t:f=w1255:i32)
            n454 = call "SetJogSpeed.vi"("Timeout (ms)"=u32 1000, "error in (no error)"=w1253, "Jog Speed"=w1252, "Motor Controller in"=w1250) -> ("error out"=w1248:errorcluster, "Motor Controller out"=w1249:refnum<class "Motor Controller.lvclass">)  [unwired: 6 in]
            n455 = Bundle By Name(cluster=T20 {"Motor Controller Parameter"=enum."Write Speed", "value"=0} ("SetExplicitMessage API Data"), "Motor Controller Parameter"=Motor_Controller_Parameter-Set."Jog Speed", "value"=w1255) -> (w1263:T20)
            n456 = Bundle By Name(cluster=T23 {"Command"=enum."GetExplicitMessage", "Arguments"="", "Data"=variant} ("API Command Cluster"), "Command"=API_Command_Enum."SetExplicitMessage", "Data"=w1263) -> (w1260:T23)
            n457 = call-dynamic "GenerateAPIEvent_Motor Controller.vi"("error in (no error)"=w1248, "API Command Cluster"=w1260, "Motor Controller In"=w1249) -> ("error out"=w1254:errorcluster)  [unwired: 6 in, 2 out]
          }
          event "Print Speed (-)": Value Change {
            n458 = event-data() -> ()  [unwired: 1 in, 6 out]
            n459 = Select(t=4999, s="Print Speed (-)", f=0) -> (s? t:f=w1269:i32)
            n460 = Unbundle By Name(w1280) -> ("Motor Controller"=w1273:refnum<class "Motor Controller.lvclass">)
            n461 = local write "Print Speed"(w1269) -> ()
            n462 = Bundle By Name(cluster=T20 {"Motor Controller Parameter"=enum."Write Speed", "value"=0} ("SetExplicitMessage API Data"), "Motor Controller Parameter"=Motor_Controller_Parameter-Set."Write Speed", "value"=w1269) -> (w1279:T20)
            n463 = Bundle By Name(cluster=T23 {"Command"=enum."GetExplicitMessage", "Arguments"="", "Data"=variant} ("API Command Cluster"), "Command"=API_Command_Enum."SetExplicitMessage", "Data"=w1279) -> (w1276:T23)
            n464 = call-dynamic "GenerateAPIEvent_Motor Controller.vi"("error in (no error)"=w1272, "API Command Cluster"=w1276, "Motor Controller In"=w1273) -> ("error out"=w1268:errorcluster)  [unwired: 6 in, 2 out]
          }
          event "Start": Value Change {
            n465 = event-data() -> ()  [unwired: 1 in, 6 out]
            n466 = Unbundle By Name(w1290) -> ("Motor Controller"=w1289:refnum<class "Motor Controller.lvclass">)
            n467 = Bundle By Name(cluster=T23 {"Command"=enum."GetExplicitMessage", "Arguments"="", "Data"=variant} ("API Command Cluster"), "Command"=API_Command_Enum."Execute Stage Move Recipe", "Data"="Stage Recipe XML File Path") -> (w1285:T23)
            n468 = call-dynamic "GenerateAPIEvent_Motor Controller.vi"("error in (no error)"=w1287, "API Command Cluster"=w1285, "Motor Controller In"=w1289) -> ("error out"=w1288:errorcluster)  [unwired: 6 in, 2 out]
          }
          event "Stage Recipe XML File Path": Value Change {
            n469 = event-data() -> ("NewVal"=w1293:path)  [unwired: 1 in, 5 out]
            n470 = Unbundle By Name(w1300) -> ("Motor Controller"=w1299:refnum<class "Motor Controller.lvclass">)
            n471 = Bundle By Name(cluster=T23 {"Command"=enum."GetExplicitMessage", "Arguments"="", "Data"=variant} ("API Command Cluster"), "Command"=API_Command_Enum."Read Stage Move Recipe", "Data"=w1293) -> (w1295:T23)
            n472 = call-dynamic "GenerateAPIEvent_Motor Controller.vi"("error in (no error)"=w1297, "API Command Cluster"=w1295, "Motor Controller In"=w1299) -> ("error out"=w1298:errorcluster)  [unwired: 6 in, 2 out]
          }
          event "Read Status": Value Change {
            n473 = event-data() -> ()  [unwired: 1 in, 6 out]
            n474 = Unbundle By Name(w1314) -> ("Motor Controller"=w1318:refnum<class "Motor Controller.lvclass">)
            n475 = Bundle By Name(cluster=T23 {"Command"=enum."GetExplicitMessage", "Arguments"="", "Data"=variant} ("API Command Cluster"), "Command"=API_Command_Enum."GetExplicitMessage", "Data"=Motor_Controller_Parameter-Get."Servo Enabled?" ("Motor Controller Parameter-Get")) -> (w1316:T23)
            n476 = call-dynamic "GenerateAPIEvent_Motor Controller.vi"("Timeout (ms)"=u32 3000, "Wait (F)"=TRUE, "error in (no error)"=w1313, "API Command Cluster"=w1316, "Motor Controller In"=w1318) -> ("error out"=w1308:errorcluster, "Return Value"=w1310:variant)  [unwired: 4 in, 1 out]
            n477 = Variant To Data(error in=w1308, type=u32 0, Variant=w1310) -> (data=w1306:u32, error out=w1307:errorcluster)
            n478 = Equal?(x=w1306, y=u32 1) -> (x = y?=w1304:bool)
            n479 = local write "Stage Enabled"(w1304) -> ()
          }
          event "Enable Ink Ch-1": Value Change {
            n480 = event-data() -> ("NewVal"=w1321:bool)  [unwired: 1 in, 5 out]
            n481 = Unbundle By Name(w1327) -> ("HeadStatusPollData.PH1_Enable"=w1326:bool)
            n482 = disable-structure shown="Enabled" {
              disable-tunnel: w1326 -> [w1338 _]
              disable-tunnel: [w1337 TRUE] -> w1325
              disable-tunnel: w1321 -> [w1336 _]
              frame Disabled {
                n483 = Not Equal?(x=w1336, y=w1338) -> (x != y?=w1337:bool)
              }
              frame Enabled {
              }
            }
            n484 = Select(t=API_Command_Enum."Enable Ink Ch-1" ("API Command"), s=w1321, f=API_Command_Enum."Disable Ink Ch-1" ("API Command")) -> (s? t:f=w1328:T26)
            n485 = Bundle By Name(cluster=w1327, "PersistentData.InkChEnable.Enable Ink Ch-1"=w1321, "API Command"=w1328) -> (w1333:T77)
            n486 = Select(t="Ink: Send Enable Command\nData: Write to Persistent File" ("State(s) in Front (\"\")"), s=w1325, f="Data: Write to Persistent File" ("State(s) in Front (\"\")")) -> (s? t:f=w1322:string)
            n487 = call <vilib>:"Add State(s) to Queue__JKI_lib_State_Machine.vi"("State(s) in Front (\"\")"=w1322, "State(s) in (\"\")"=w1331) -> ("States Out"=w1332:string)  [unwired: 13 in]
          }
          event "Enable Ink Ch-2": Value Change {
            n488 = event-data() -> ("NewVal"=w1342:bool)  [unwired: 1 in, 5 out]
            n489 = Unbundle By Name(w1341) -> ("HeadStatusPollData.PH2_Enable"=w1346:bool)
            n490 = disable-structure shown="Enabled" {
              disable-tunnel: w1346 -> [w1357 _]
              disable-tunnel: [w1356 TRUE] -> w1345
              disable-tunnel: w1342 -> [w1355 _]
              frame Disabled {
                n491 = Not Equal?(x=w1355, y=w1357) -> (x != y?=w1356:bool)
              }
              frame Enabled {
              }
            }
            n492 = Select(t=API_Command_Enum."Enable Ink Ch-2" ("API Command"), s=w1342, f=API_Command_Enum."Disable Ink Ch-2" ("API Command")) -> (s? t:f=w1347:T26)
            n493 = Bundle By Name(cluster=w1341, "PersistentData.InkChEnable.Enable Ink Ch-2"=w1342, "API Command"=w1347) -> (w1352:T77)
            n494 = Select(t="Ink: Send Enable Command\nData: Write to Persistent File" ("State(s) in Front (\"\")"), s=w1345, f="Data: Write to Persistent File" ("State(s) in Front (\"\")")) -> (s? t:f=w1340:string)
            n495 = call <vilib>:"Add State(s) to Queue__JKI_lib_State_Machine.vi"("State(s) in Front (\"\")"=w1340, "State(s) in (\"\")"=w1350) -> ("States Out"=w1351:string)  [unwired: 13 in]
          }
          event "Enable Ink Ch-3": Value Change {
            n496 = event-data() -> ("NewVal"=w1360:bool)  [unwired: 1 in, 5 out]
            n497 = Unbundle By Name(w1361) -> ("HeadStatusPollData.PH3_Enable"=w1365:bool)
            n498 = disable-structure shown="Enabled" {
              disable-tunnel: w1365 -> [w1376 _]
              disable-tunnel: [w1375 TRUE] -> w1364
              disable-tunnel: w1360 -> [w1374 _]
              frame Disabled {
                n499 = Not Equal?(x=w1374, y=w1376) -> (x != y?=w1375:bool)
              }
              frame Enabled {
              }
            }
            n500 = Select(t=API_Command_Enum."Enable Ink Ch-3" ("API Command"), s=w1360, f=API_Command_Enum."Disable Ink Ch-3" ("API Command")) -> (s? t:f=w1366:T26)
            n501 = Bundle By Name(cluster=w1361, "PersistentData.InkChEnable.Enable Ink Ch-3"=w1360, "API Command"=w1366) -> (w1371:T77)
            n502 = Select(t="Ink: Send Enable Command\nData: Write to Persistent File" ("State(s) in Front (\"\")"), s=w1364, f="Data: Write to Persistent File" ("State(s) in Front (\"\")")) -> (s? t:f=w1359:string)
            n503 = call <vilib>:"Add State(s) to Queue__JKI_lib_State_Machine.vi"("State(s) in Front (\"\")"=w1359, "State(s) in (\"\")"=w1369) -> ("States Out"=w1370:string)  [unwired: 13 in]
          }
          event "Enable Ink Ch-4": Value Change {
            n504 = event-data() -> ("NewVal"=w1379:bool)  [unwired: 1 in, 5 out]
            n505 = Unbundle By Name(w1380) -> ("HeadStatusPollData.PH4_Enable"=w1384:bool)
            n506 = disable-structure shown="Enabled" {
              disable-tunnel: w1384 -> [w1395 _]
              disable-tunnel: [w1394 TRUE] -> w1383
              disable-tunnel: w1379 -> [w1393 _]
              frame Disabled {
                n507 = Not Equal?(x=w1393, y=w1395) -> (x != y?=w1394:bool)
              }
              frame Enabled {
              }
            }
            n508 = Select(t=API_Command_Enum."Enable Ink Ch-4" ("API Command"), s=w1379, f=API_Command_Enum."Disable Ink Ch-4" ("API Command")) -> (s? t:f=w1385:T26)
            n509 = Bundle By Name(cluster=w1380, "PersistentData.InkChEnable.Enable Ink Ch-4"=w1379, "API Command"=w1385) -> (w1390:T77)
            n510 = Select(t="Ink: Send Enable Command\nData: Write to Persistent File" ("State(s) in Front (\"\")"), s=w1383, f="Data: Write to Persistent File" ("State(s) in Front (\"\")")) -> (s? t:f=w1378:string)
            n511 = call <vilib>:"Add State(s) to Queue__JKI_lib_State_Machine.vi"("State(s) in Front (\"\")"=w1378, "State(s) in (\"\")"=w1388) -> ("States Out"=w1389:string)  [unwired: 13 in]
          }
          event "Enable Ink Ch-5": Value Change {
            n512 = event-data() -> ("NewVal"=w1398:bool)  [unwired: 1 in, 5 out]
            n513 = Unbundle By Name(w1399) -> ("HeadStatusPollData.PH5_Enable"=w1403:bool)
            n514 = disable-structure shown="Enabled" {
              disable-tunnel: w1403 -> [w1414 _]
              disable-tunnel: [w1413 TRUE] -> w1402
              disable-tunnel: w1398 -> [w1412 _]
              frame Disabled {
                n515 = Not Equal?(x=w1412, y=w1414) -> (x != y?=w1413:bool)
              }
              frame Enabled {
              }
            }
            n516 = Select(t=API_Command_Enum."Enable Ink Ch-5" ("API Command"), s=w1398, f=API_Command_Enum."Disable Ink Ch-5" ("API Command")) -> (s? t:f=w1404:T26)
            n517 = Bundle By Name(cluster=w1399, "PersistentData.InkChEnable.Enable Ink Ch-5"=w1398, "API Command"=w1404) -> (w1409:T77)
            n518 = Select(t="Ink: Send Enable Command\nData: Write to Persistent File" ("State(s) in Front (\"\")"), s=w1402, f="Data: Write to Persistent File" ("State(s) in Front (\"\")")) -> (s? t:f=w1397:string)
            n519 = call <vilib>:"Add State(s) to Queue__JKI_lib_State_Machine.vi"("State(s) in Front (\"\")"=w1397, "State(s) in (\"\")"=w1407) -> ("States Out"=w1408:string)  [unwired: 13 in]
          }
          event "Enable Ink Ch-6": Value Change {
            n520 = event-data() -> ("NewVal"=w1417:bool)  [unwired: 1 in, 5 out]
            n521 = Unbundle By Name(w1418) -> ("HeadStatusPollData.PH6_Enable"=w1422:bool)
            n522 = disable-structure shown="Enabled" {
              disable-tunnel: w1422 -> [w1433 _]
              disable-tunnel: [w1432 TRUE] -> w1421
              disable-tunnel: w1417 -> [w1431 _]
              frame Disabled {
                n523 = Not Equal?(x=w1431, y=w1433) -> (x != y?=w1432:bool)
              }
              frame Enabled {
              }
            }
            n524 = Select(t=API_Command_Enum."Enable Ink Ch-6" ("API Command"), s=w1417, f=API_Command_Enum."Disable Ink Ch-6" ("API Command")) -> (s? t:f=w1423:T26)
            n525 = Bundle By Name(cluster=w1418, "PersistentData.InkChEnable.Enable Ink Ch-6"=w1417, "API Command"=w1423) -> (w1428:T77)
            n526 = Select(t="Ink: Send Enable Command\nData: Write to Persistent File" ("State(s) in Front (\"\")"), s=w1421, f="Data: Write to Persistent File" ("State(s) in Front (\"\")")) -> (s? t:f=w1416:string)
            n527 = call <vilib>:"Add State(s) to Queue__JKI_lib_State_Machine.vi"("State(s) in Front (\"\")"=w1416, "State(s) in (\"\")"=w1426) -> ("States Out"=w1427:string)  [unwired: 13 in]
          }
          event "StartPrime 1", "StartPrime 2", "StartPrime 3", "StartPrime 4", "StartPrime 5", "StartPrime 6": Value Change {
            w1439 = T27 {"Interval (s)"=0.1, "PurgeDuration (s)"=0.1, "Repeats"=0, "PrimingMode"=enum."Pre-Purge", "Head"=enum."-1", "Frequency (Hz)"=0, "PrintWeight"=0.1} ("Pre Purge API Data")
            n528 = event-data() -> ("CtlRef"=w1447:refnum<vi>)  [unwired: 1 in, 5 out]
            n529 = property class="Bool"(reference=w1447) -> ("Label.Text"=w1446:string)  [unwired: 1 in, 2 out]
            n530 = case shown="\"StartPrime 6\", \"StartPrime1 6\"" w1446 {
              tunnel: w1445 -> [_ w1455 w1457 w1459 w1461 w1463 w1465]
              tunnel: ["" w1454 w1456 w1458 w1460 w1462 w1464] -> w1440
              frame Default {
              }
              frame "StartPrime 1", "StartPrime1 1" {
                n531 = Unbundle By Name(w1455) -> ("Prime Names.Prime 1"=w1454:string)
              }
              frame "StartPrime 2", "StartPrime1 2" {
                n532 = Unbundle By Name(w1457) -> ("Prime Names.Prime 2"=w1456:string)
              }
              frame "StartPrime 3", "StartPrime1 3" {
                n533 = Unbundle By Name(w1459) -> ("Prime Names.Prime 3"=w1458:string)
              }
              frame "StartPrime 4", "StartPrime1 4" {
                n534 = Unbundle By Name(w1461) -> ("Prime Names.Prime 4"=w1460:string)
              }
              frame "StartPrime 5", "StartPrime1 5" {
                n535 = Unbundle By Name(w1463) -> ("Prime Names.Prime 5"=w1462:string)
              }
              frame "StartPrime 6", "StartPrime1 6" {
                n536 = Unbundle By Name(w1465) -> ("Prime Names.Prime 6"=w1464:string)
              }
            }
            n537 = Unbundle By Name(w1445) -> ("TopLevel out"=w1441:refnum<class "TopLevel.lvclass">)
            n538 = call-dynamic "Read ConfigDict.vi"("error in (no error)"=w1436, "TopLevel in"=w1441) -> ("error out"=w1437:errorcluster, "ConfigDIct"=w1444:T16)  [unwired: 7 in, 1 out]
            n539 = call <vilib>:"Get Dynamic CVT Data.vi"("error in (no error)"=w1437, "default value (empty variant)"=w1439, "DataName"=w1440, "dCVT DVR"=w1444) -> ("error out"=w1443:errorcluster, "value"=w1442:variant)  [unwired: 4 in, 2 out]
            n540 = Variant To Data(error in=w1443, type=w1439, Variant=w1442) -> (data=w1438:T27, error out=w1435:errorcluster)
            n541 = Bundle By Name(cluster=w1445, "Pre Purge API Data"=w1438) -> (w1448:T77)
            n542 = call <vilib>:"Add State(s) to Queue__JKI_lib_State_Machine.vi"("State(s) in Front (\"\")"="Prime: Send API", "State(s) in (\"\")"=w1450) -> ("States Out"=w1451:string)  [unwired: 13 in]
          }
          event "Stage Head1 2", "Stage Head2 2", "Stage Head3 2", "Stage Head4 2", "Stage Head5 2", "Stage Head6 2": Value Change {
            w1483 = T27 {"Interval (s)"=0.1, "PurgeDuration (s)"=0.1, "Repeats"=0, "PrimingMode"=enum."Pre-Purge", "Head"=enum."1", "Frequency (Hz)"=0, "PrintWeight"=0.1} ("Pre Purge API Data")
            n543 = event-data() -> ("CtlRef"=w1491:refnum<vi>)  [unwired: 1 in, 5 out]
            n544 = property class="Bool"(reference=w1491, error in=w1490) -> (error out=w1486:errorcluster, "Label.Text"=w1489:string)  [unwired: 1 out]
            n545 = case shown="\"Stage Head3\", \"Stage Head3 2\"" w1489 {
              tunnel: w1488 -> [w1498 w1503 w1508 w1513 w1518 w1523]
              tunnel: [w1497 w1502 w1507 w1512 w1517 w1522] -> w1485
              tunnel: [Motor_Controller_Parameter-Set."Move Stage to Under PH1" ("Motor Controller Parameter") Motor_Controller_Parameter-Set."Move Stage to Under PH2" ("Motor Controller Parameter") Motor_Controller_Parameter-Set."Move Stage to Under PH3" ("Motor Controller Parameter") Motor_Controller_Parameter-Set."Move Stage to Under PH4" ("Motor Controller Parameter") Motor_Controller_Parameter-Set."Move Stage to Under PH5" ("Motor Controller Parameter") Motor_Controller_Parameter-Set."Move Stage to Under PH6" ("Motor Controller Parameter")] -> w1471
              tunnel: [4 ("value") 5 ("value") 6 ("value") 7 ("value") 8 ("value") 9 ("value")] -> w1468
              tunnel: [11 ("value") 12 ("value") 13 ("value") 14 ("value") 15 ("value") 16 ("value")] -> w1467
              frame "Stage Head1", "Stage Head1 2", Default {
                n546 = Unbundle By Name(w1498) -> ("Prime Names.Prime 1"=w1497:string)
              }
              frame "Stage Head2", "Stage Head2 2" {
                n547 = Unbundle By Name(w1503) -> ("Prime Names.Prime 2"=w1502:string)
              }
